vi "Panel.vi"(11 "PlatformListPanel in":refnum<class "PlatformListPanel.lvclass">) -> ()   [LabVIEW 2020, in "PicoG-App.lvlib" / "PlatformListPanel.lvclass"]
uses:
  PlatformListPanel.lvclass
  C:/Program Files (x86)/National Instruments/LabVIEW 2020/vi.lib/IlluminatedG/IG OOPanel/OOPanel/Panel/Panel.lvclass
  <vilib>/IlluminatedG/IG OOPanel/OOPanel/Panel/Basic UI State.ctl
  PlatformArrayPanel/PlatformArrayPanel.lvclass
  C:/Program Files (x86)/National Instruments/LabVIEW 2020/vi.lib/IlluminatedG/IG OOPanel/OOPanel/ArrayPanel/ArrayPanel.lvclass
  PlatformListPanel.lvclass/PlatformListPanel.ctl
  <vilib>/IlluminatedG/IG OOPanel/OOPanel/Panel/Panel.lvclass
  <vilib>/IlluminatedG/IG OOPanel/OOPanel/OOPanel.lvlib
  Builds/picoG/ppl/PicoG-Core.lvlibp/PicoG-Processor/PicoG-Core/PlatformPluginManager/PlatformPluginManager.lvclass
  <vilib>/IlluminatedG/IG OOPanel/OOPanel/ArrayManager/ArrayManager.lvclass
panel:
  # "These are the platform plugins that were loaded at startup. Adding new plugins requires restarting the picoG application."
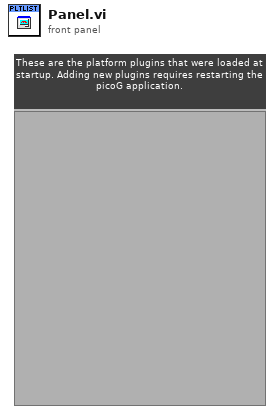
[diagram p1: front panel]
types:
  T1 = typedef "OOPanel.lvlib/Panel.lvclass/Basic UI State.ctl" = enum16{"Init", "Run", "Close"}
  T2 = typedef "OOPanel.lvlib/Panel.lvclass/Panel Events.ctl" = cluster{"Visbility":refnum<user-event>, "Close":refnum<user-event>}
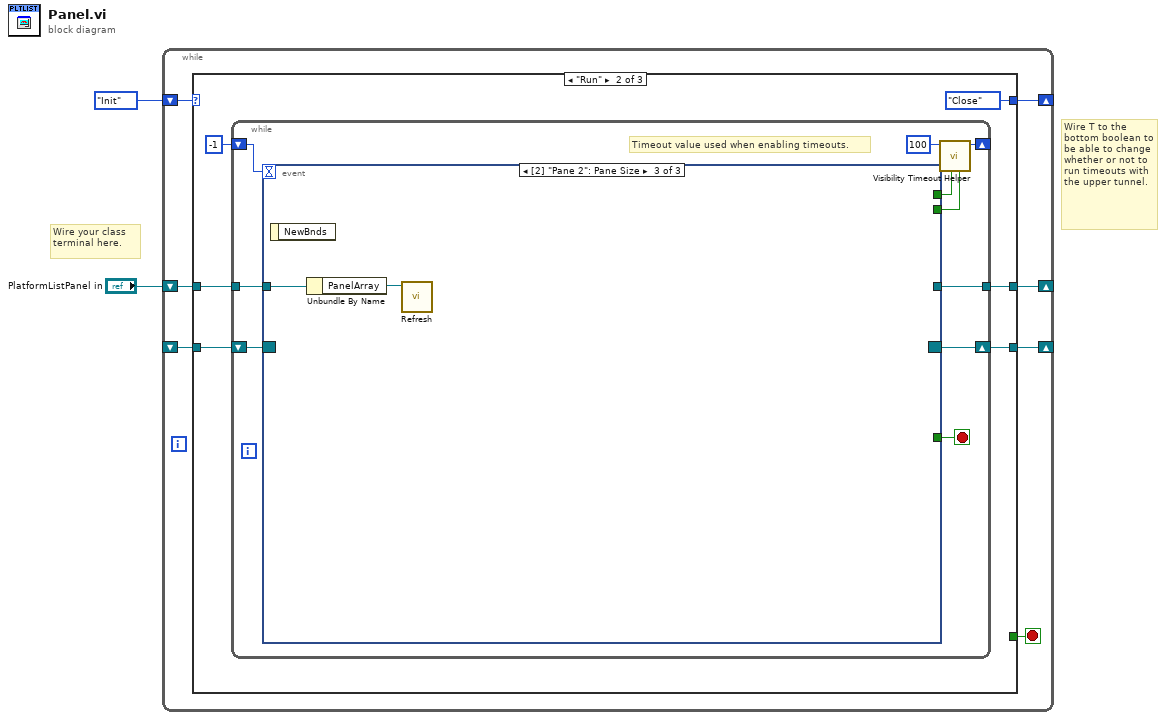
[diagram p0: block diagram]
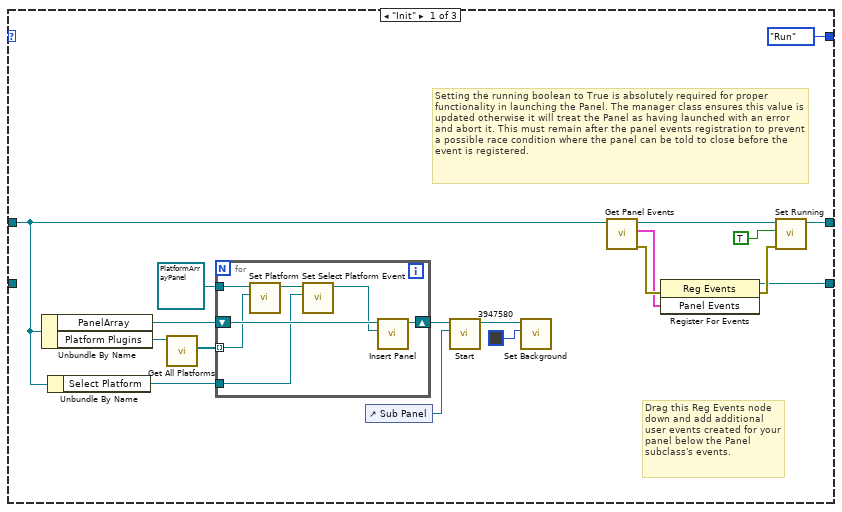
[diagram p2: hidden frame]
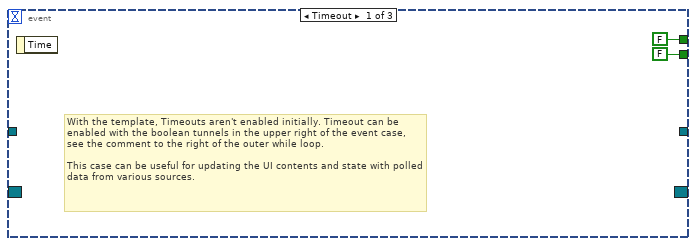
[diagram p3: hidden frame]
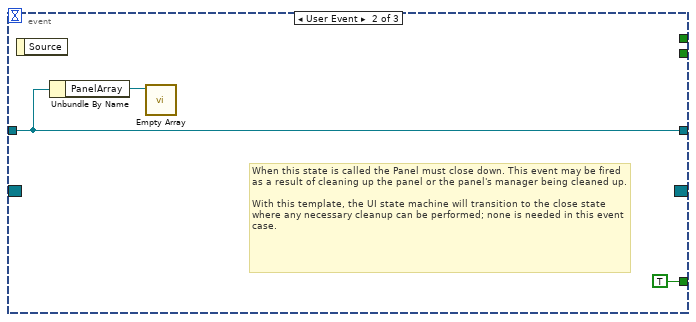
[diagram p4: hidden frame]
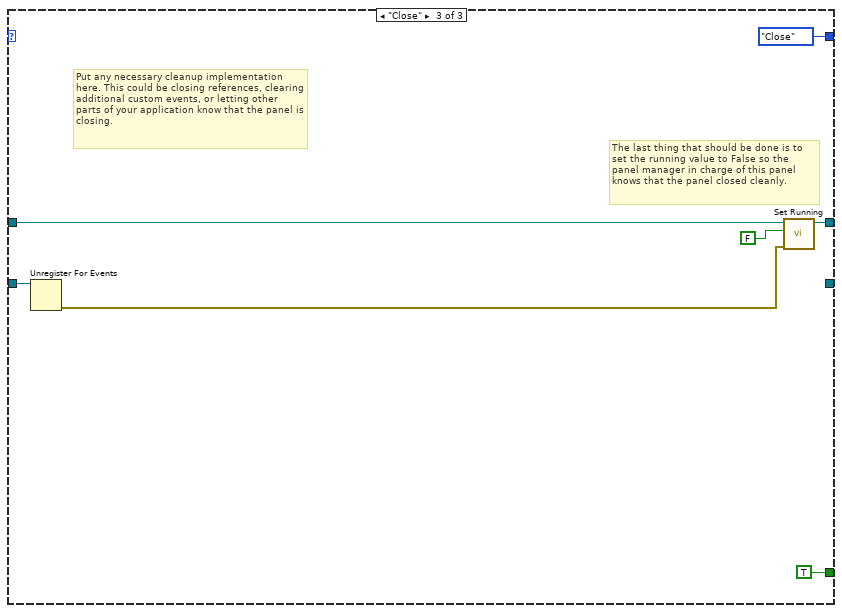
[diagram p5: hidden frame]
diagram:
  # "Wire T to the bottom boolean to be able to change whether or not to run timeouts with the upper tunnel."
  # "Wire your class terminal here."
  n1 = while {
    shift-right: [w8] -> _
    shift-left: _ -> [w9]
    shift-right: [w6] -> _
    shift-left: Basic_UI_State."Init" ("Basic UI State") -> [w7]
    shift-right: [w4] -> _
    shift-left: "PlatformListPanel in" -> [w3]
    stop <- w5 stop-if-true
    n2 = case shown="\"Run\"" w7 {
      tunnel: w9 -> [_ w40 w60]
      tunnel: [w21 w38 _] -> w8
      tunnel: [Basic_UI_State."Run" ("Basic UI State") Basic_UI_State."Close" ("Basic UI State") Basic_UI_State."Close" ("Basic UI State")] -> w6
      tunnel: [_ _ TRUE] -> w5
      tunnel: [w20 w35 w58] -> w4
      tunnel: w3 -> [w13 w36 w59]
      frame "Init" {
        # "Setting the running boolean to True is absolutely required for proper functionality in launching the Panel. The manager class ensures this value is updated otherwise it will treat the Panel as having launched with an error and abort it. This must remain after the panel events registration to prevent a possible race condition where the panel can be told to close before the event is registered."
        # "Drag this Reg Events node down and add additional user events created for your panel below the Panel subclass's events."
        n3 = Unbundle By Name(w13) -> ("PanelArray"=w17:refnum<class "ArrayManager.lvclass">, "Platform Plugins"=w19:refnum<class "PlatformPluginManager.lvclass">)
        n4 = Unbundle By Name(w13) -> ("Select Platform"=w12:refnum<user-event>)
        n5 = call "Get All Platforms.vi"("TargetPluginManager in"=w19) -> ("Platforms"=w18:refnum<class "DeployPlatform.lvclass">[])  [unwired: 8 in, 2 out]
        n6 = for {
          tunnel: w18 -> [w31] mode=indexing
          shift-right: [w32] -> w15
          shift-left: w17 -> [w34]
          tunnel: refnum<class "PlatformArrayPanel.lvclass"> refnum ("PicoG-App.lvlib:PlatformArrayPanel.lvclass") -> [w33]
          tunnel: w12 -> [w29]
          n7 = call "Set Platform.vi"("Platform"=w31, "PlatformArrayPanel in"=w33) -> ("PlatformArrayPanel out"=w30:refnum<class "PlatformArrayPanel.lvclass">)  [unwired: 8 in, 1 out]
          n8 = call "Set Select Platform Event.vi"("Select Platform Event"=w29, "PlatformArrayPanel in"=w30) -> ("PlatformArrayPanel out"=w28:refnum<class "PlatformArrayPanel.lvclass">)  [unwired: 8 in, 1 out]
          n9 = call <vilib>:"Insert Panel.vi"("Panel/Type"=w28, "PanelArray in"=w34) -> ("PanelArray out"=w32:refnum<class "ArrayManager.lvclass">)  [unwired: 7 in, 2 out]
        }
        n10 = control-ref of="Sub Panel"() -> (w14:refnum<vi>)
        n11 = call <vilib>:"Start.vi"("Container"=w14, "ArrayManager in"=w15) -> ("ArrayManager out"=w10:refnum<class "ArrayManager.lvclass">)  [unwired: 8 in, 1 out]
        n12 = call <vilib>:"Set Background.vi"("Background"=u32 3947580, "ArrayManager in"=w10) -> ()  [unwired: 8 in, 2 out]
        n13 = call <vilib>:"Get Panel Events.vi"("Panel in"=w13) -> ("error out"=w27:errorcluster, "Panel Events"=w23:T2, "Panel out"=w24:refnum<class "PlatformListPanel.lvclass">)  [unwired: 8 in]
        n14 = register-events(error in=w27, w23) -> (reference out=w21:refnum<event-registration>, error out=w25:errorcluster)  [unwired: 1 in]
        n15 = call <vilib>:"Set Running.vi"("error in (no error)"=w25, "Running"=TRUE, "Panel in"=w24) -> ("Panel out"=w20:refnum<class "PlatformListPanel.lvclass">)  [unwired: 7 in, 1 out]
      }
      frame "Run" {
        n16 = while {
          shift-right: [w46] -> w38
          shift-left: w40 -> [w47]
          shift-right: [w49] -> _
          shift-left: -1 ("Timeout") -> [w48]
          tunnel: w36 -> [w42]
          tunnel: [w41] -> w35
          stop <- w43 stop-if-true
          # "Timeout value used when enabling timeouts."
          n17 = event shown="[2] \"Pane 2\": Pane Size" {
            selector: w47 -> [_ _ _]
            dyn-events: [_ _ _] -> w46
            timeout: w48 -> [_ _ _]
            tunnel: [FALSE _ _] -> w45
            tunnel: [FALSE _ _] -> w44
            tunnel: [_ TRUE _] -> w43
            tunnel: w42 -> [_ w54 w56]
            tunnel: [_ w54 _] -> w41
            event Timeout {
              # "With the template, Timeouts aren't enabled initially. Timeout can be enabled with the boolean tunnels in the upper right of the event case, see the comment to the right of the outer while loop.\n\nThis case can be useful for updating the UI contents and state with polled data from various sources."
              n18 = event-data() -> ()  [unwired: 1 in, 1 out]
            }
            event User Event {
              # "When this state is called the Panel must close down. This event may be fired as a result of cleaning up the panel or the panel's manager being cleaned up.\n\nWith this template, the UI state machine will transition to the close state where any necessary cleanup can be performed; none is needed in this event case."
              n19 = event-data() -> ()  [unwired: 1 in, 1 out]
              n20 = Unbundle By Name(w54) -> ("PanelArray"=w53:refnum<class "ArrayManager.lvclass">)
              n21 = call <vilib>:"Empty Array.vi"("ArrayManager in"=w53) -> ()  [unwired: 9 in, 2 out]
            }
            event Pane Size {
              n22 = event-data() -> ()  [unwired: 1 in, 1 out]
              n23 = Unbundle By Name(w56) -> ("PanelArray"=w57:refnum<class "ArrayManager.lvclass">)
              n24 = call <vilib>:"Refresh.vi"("ArrayManager in"=w57) -> ()  [unwired: 9 in, 2 out]
            }
          }
          n25 = call <vilib>:"Visibility Timeout Helper.vi"("Update?"=w44, "Use Timeout?"=w45, "Visible Timeout mS"=100) -> ("Timeout"=w49:i32)  [unwired: 8 in]
        }
      }
      frame "Close" {
        # "Put any necessary cleanup implementation here. This could be closing references, clearing additional custom events, or letting other parts of your application know that the panel is closing."
        # "The last thing that should be done is to set the running value to False so the panel manager in charge of this panel knows that the panel closed cleanly."
        n26 = Unregister For Events(event registration refnum=w60) -> (error out=w62:errorcluster)  [unwired: 1 in]
        n27 = call <vilib>:"Set Running.vi"("error in (no error)"=w62, "Running"=FALSE, "Panel in"=w59) -> ("Panel out"=w58:refnum<class "PlatformListPanel.lvclass">)  [unwired: 7 in, 1 out]
      }
    }
  }
